vi "MacroGUI_MD.vi"() -> ()   [LabVIEW 2012]
uses:
  Custom Controls and Typedefs/Available Operations Tree.ctl
  Custom Controls and Typedefs/Edit Button.ctl
  Custom Controls and Typedefs/Delete Button.ctl
  Custom Controls and Typedefs/TimeUpdate.ctl
  Custom Controls and Typedefs/Macro_MD_UI Control Refnums.ctl
  Custom Controls and Typedefs/MacroExecutionStates.ctl
  SubVIs/FGV_MacroGen_Commands.ctl
  Custom Controls and Typedefs/Macro_CommandStruct.ctl
  Custom Controls and Typedefs/Macro_Action_List.ctl
  Custom Controls and Typedefs/Macro_ArgumentStruct.ctl
  SubVIs/FormatTree&TableStyle_Commands.ctl
  SubVIs/Timer_MacroGen_Commands.ctl
  <vilib>/Utility/file.llb/Write To Spreadsheet File (string).vi
  GFG/GFG library.lvlib
panel:
  out "Status":string
  out "Index":i32
  out "Timing Data":T1 {"Seconds" scale=0.0..60.0}
  in  "MacroTreeOperation":T4
  in  "File Operation Cluster":cluster{"Load Macro":bool, "SaveAs":bool}
  in  "Table Navigation Cluster":T5
  in  "Parameters":string[][](table)
  in  "Execute Macro":bool
  in  "Add":bool
  in  "Available Actions":T6
  in  "stop":bool
  in  "Macro":string(tree)
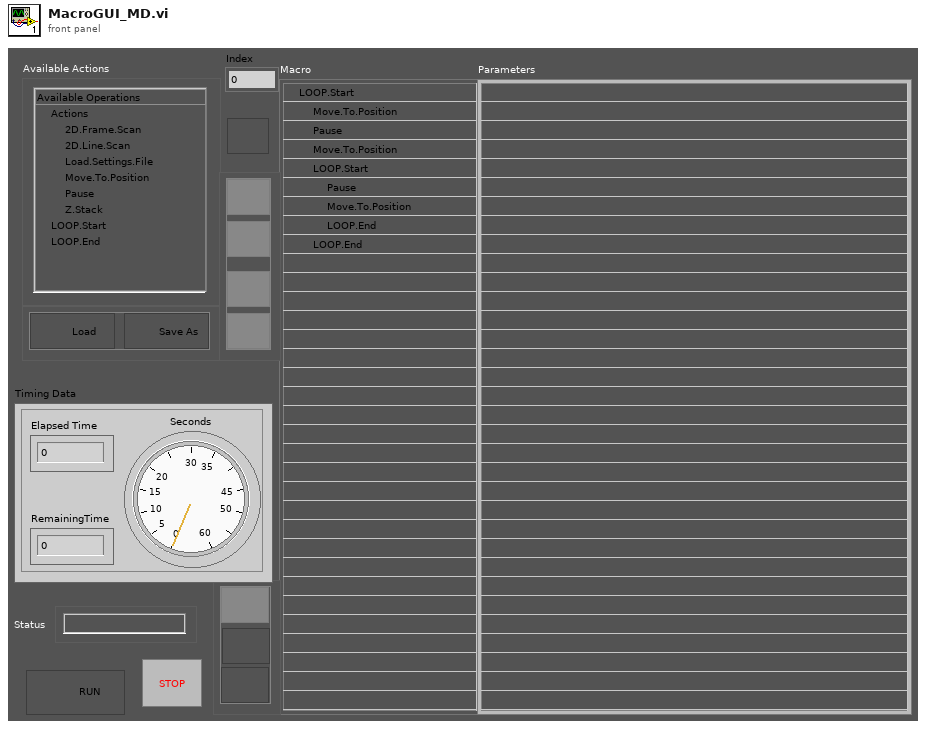
[diagram p1: front panel]
types:
  T1 = typedef "TimeUpdate.ctl" = cluster{"Seconds":dbl, "Elapsed Time":dbl, "RemainingTime":dbl}
  T2 = typedef "Edit Button.ctl" = bool
  T3 = typedef "Delete Button.ctl" = bool
  T4 = cluster{"Save Button":bool, "Edit Button":T2, "Delete Button":T3}
  T5 = cluster{"Table Index Up":bool, "Table Index Up-End":bool, "Table Index Down":bool, "Table Index Down-End":bool}
  T6 = typedef "Available Operations Tree.ctl" = string
  T7 = typedef "MacroExecutionStates.ctl" = enum16{"UI Mode", "Execute Command", "Wait for completion", "Pause"}
  T8 = typedef "Macro_MD_UI Control Refnums.ctl" = cluster{"Available Operations":refnum<vi>, "Created Macro":refnum<vi>, "Indent Item":refnum<vi>, "Add Selected to Macro":refnum<vi>, "Outdent Item":refnum<vi>, "Number of Iterations":refnum<vi>, "Seconds to Wait":refnum<vi>, "Load Macro":refnum<vi>, "Save Macro":refnum<vi>, "Select File to Load":refnum<vi>, "Params Table":refnum<vi>, "Delete":refnum<vi>, "Edit Button":refnum<vi>, "Execute Macro":refnum<vi>}
  T9 = typedef "FGV_MacroGen_Commands.ctl" = enum16{"Initialize", "Get Array", "Load from file", "Insert Item", "Insert at End", "Edit Item", "Delete Item", "Move Items", "Save", "SaveAs"}
  T10 = typedef "FormatTree&TableStyle_Commands.ctl" = enum16{"Colour Row", "Uncolour Row", "Bold Row", "Unbold Row", "Clear", "UpdateVisibleRows"}
  T11 = typedef "Macro_CommandStruct.ctl" = cluster{"Action":T12, "Arguments":T13[]}
  T12 = typedef "Macro_Action_List.ctl" = enum16{"Unknown", "2D.Frame.Scan", "2D.Line.Scan", "Load.Settings.File", "Move.To.Position", "Pause", "Z.Stack", "LOOP.Start", "LOOP.End"}
  T13 = typedef "Macro_ArgumentStruct.ctl" = cluster{"ArgumentName":string, "DataType":enum16{"Numeric", "String"}, "Value":variant}
  T14 = typedef "Timer_MacroGen_Commands.ctl" = enum16{"Start", "Pause", "Run"}
  T15 = cluster{"data name":string, "drag data":variant}[]
  T16 = typedef "LVPoint32TypeDef.ctl" = cluster{"Horizontal":i32, "Vertical":i32}
  T17 = typedef "LVRowAndColumnTypeDef.ctl" = cluster{"Row":i32, "Column":i32}
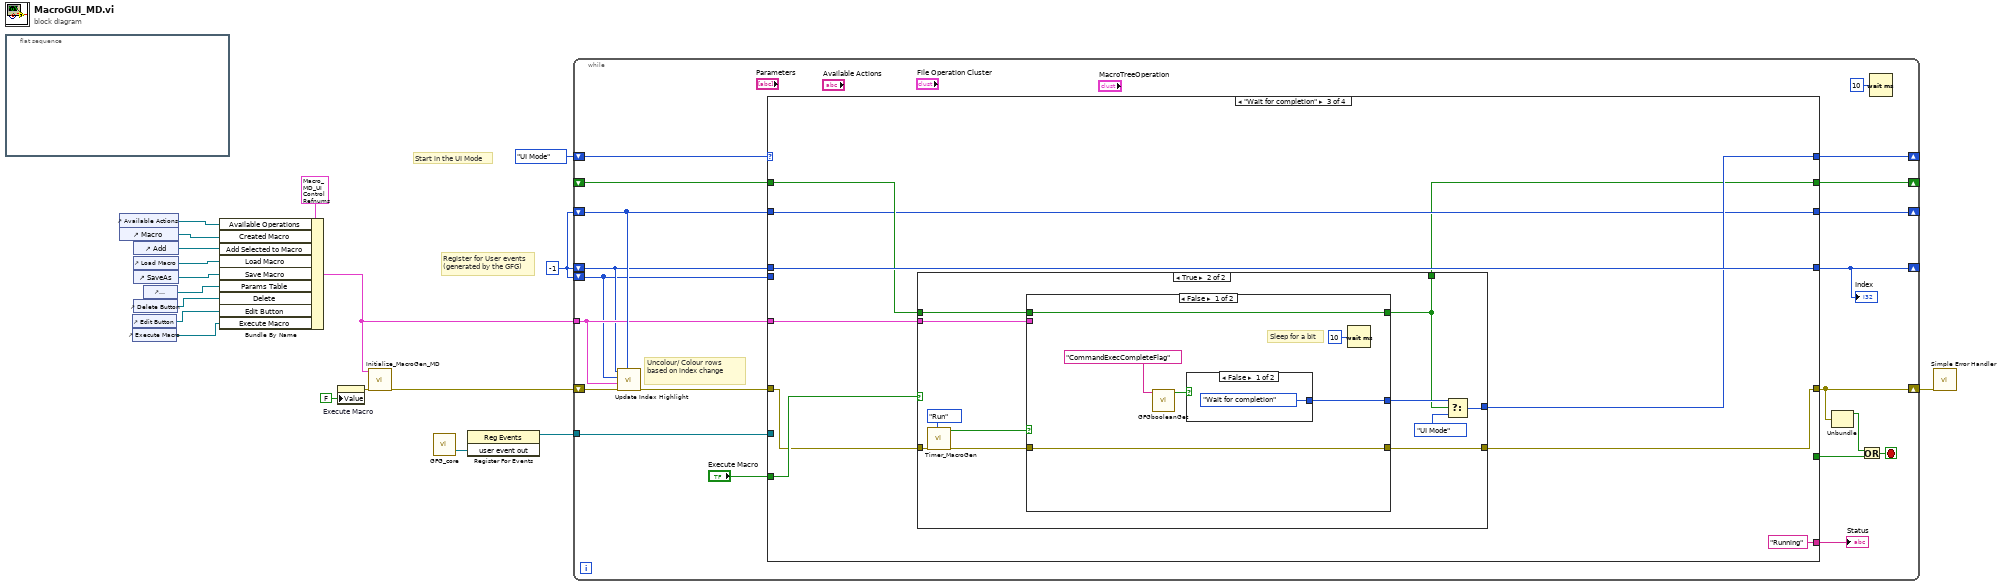
[diagram p0: block diagram]
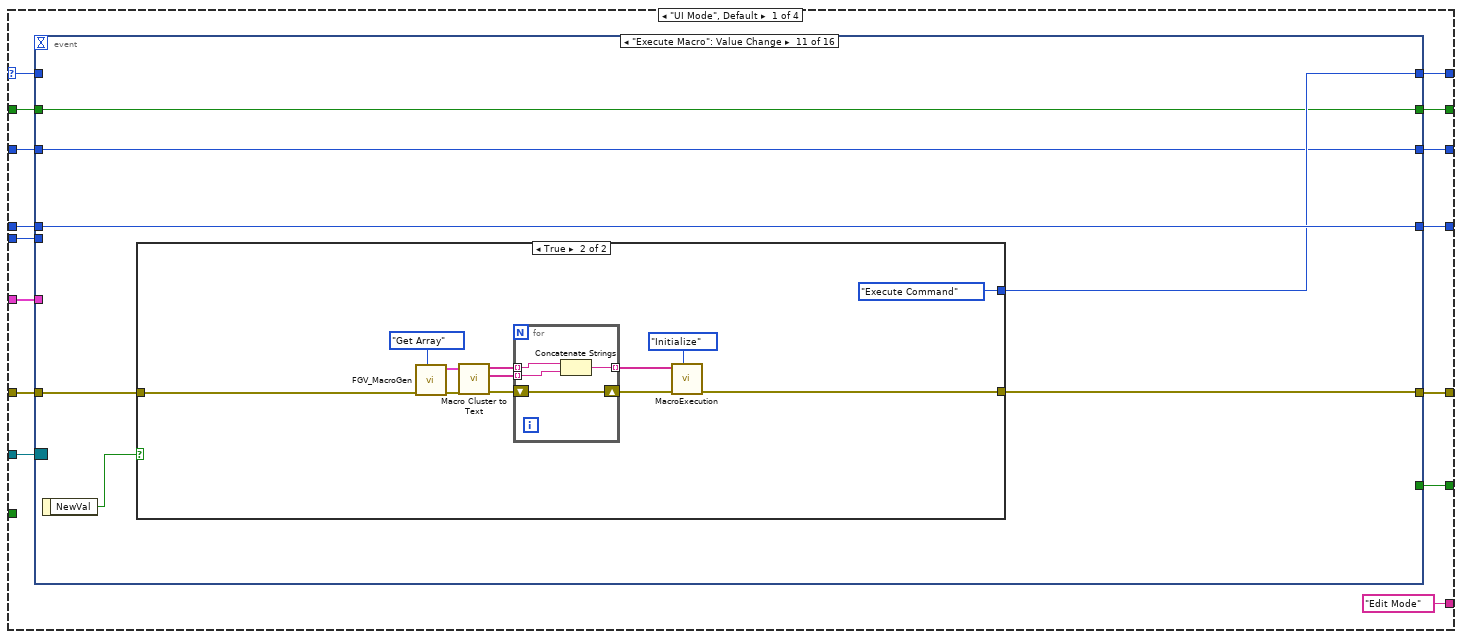
[diagram p2: hidden frame]
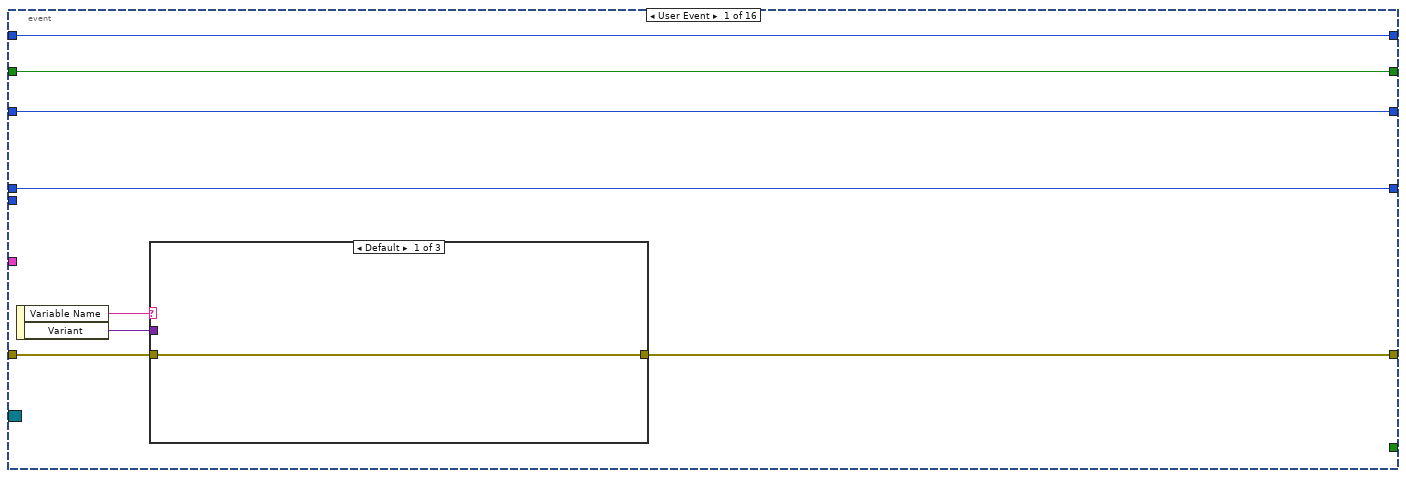
[diagram p3: hidden frame]
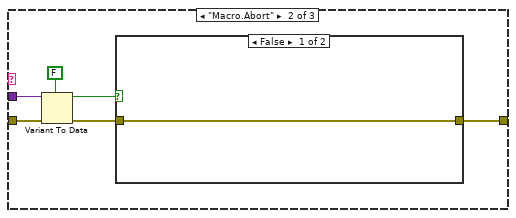
[diagram p4: hidden frame]
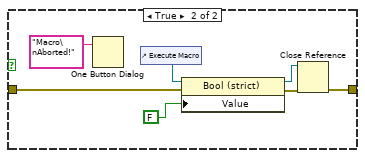
[diagram p5: hidden frame]
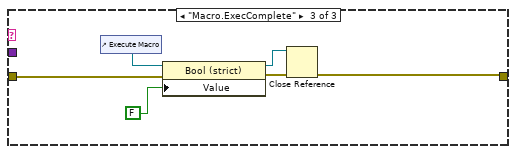
[diagram p6: hidden frame]
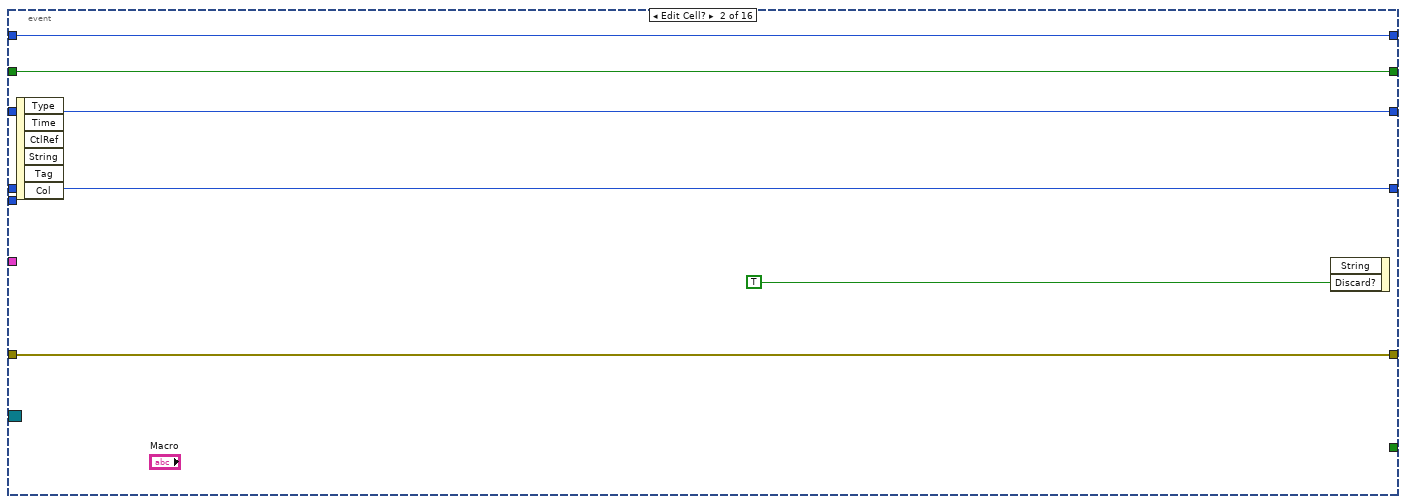
[diagram p7: hidden frame]
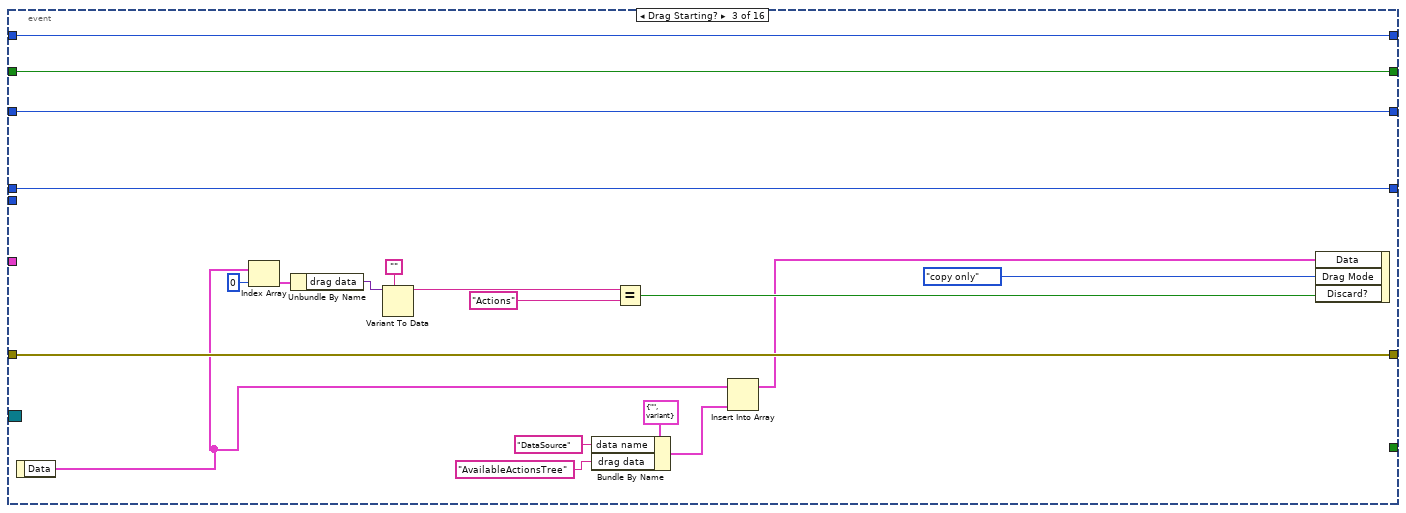
[diagram p8: hidden frame]
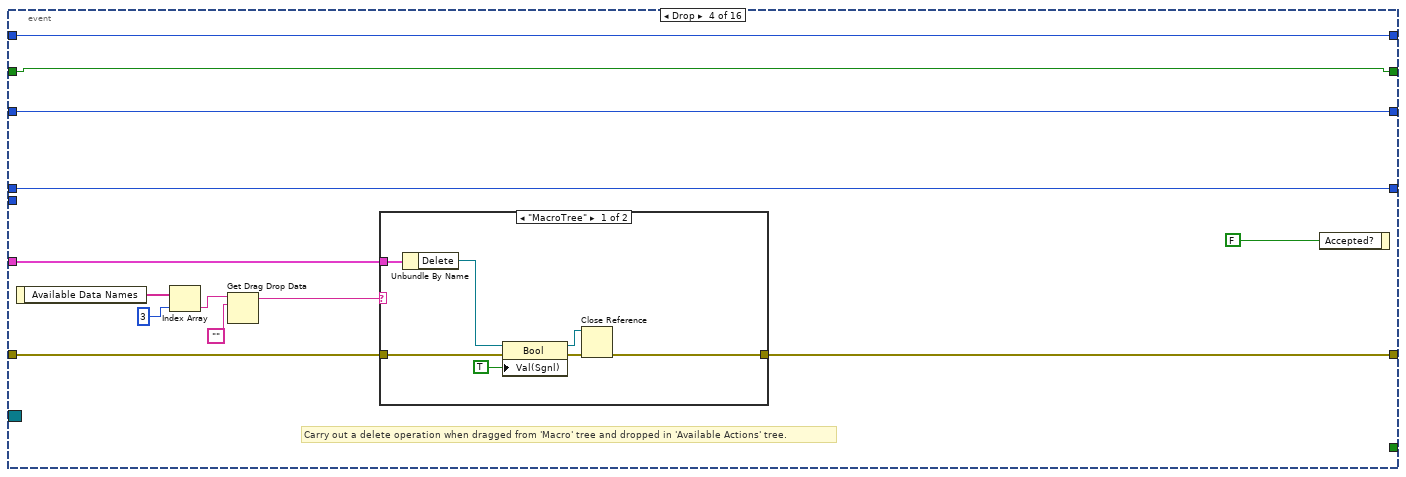
[diagram p9: hidden frame]
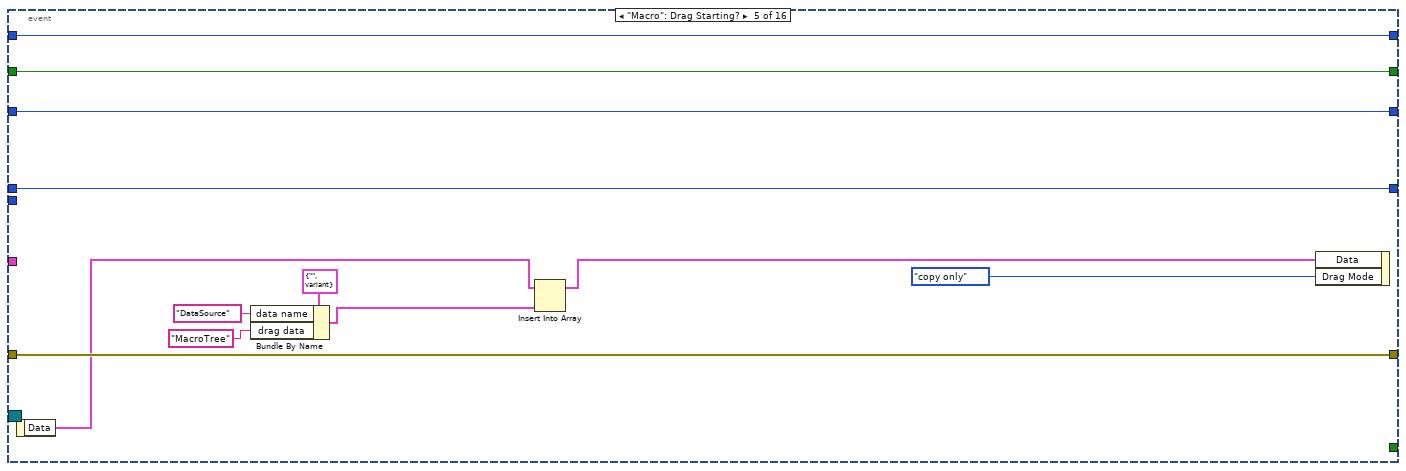
[diagram p11: hidden frame]
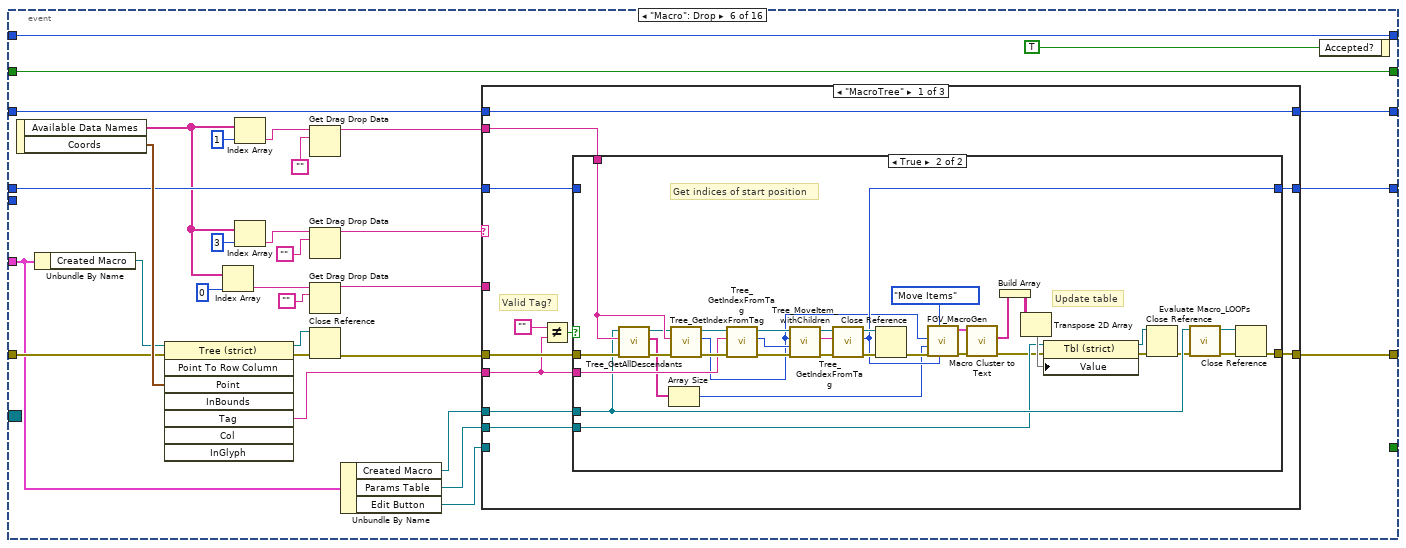
[diagram p12: hidden frame]
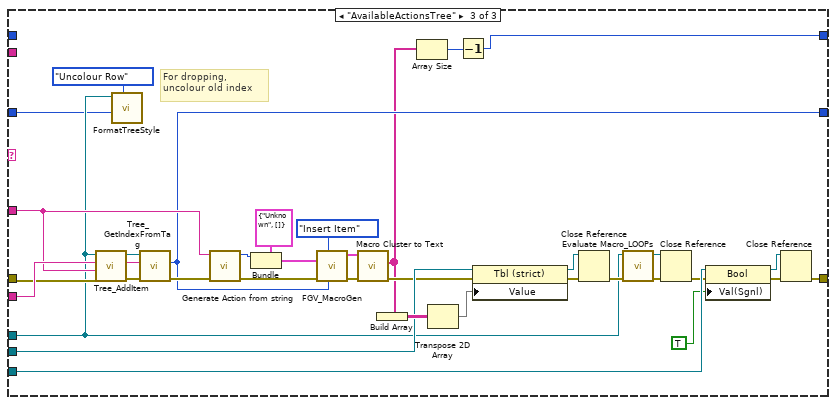
[diagram p15: hidden frame]
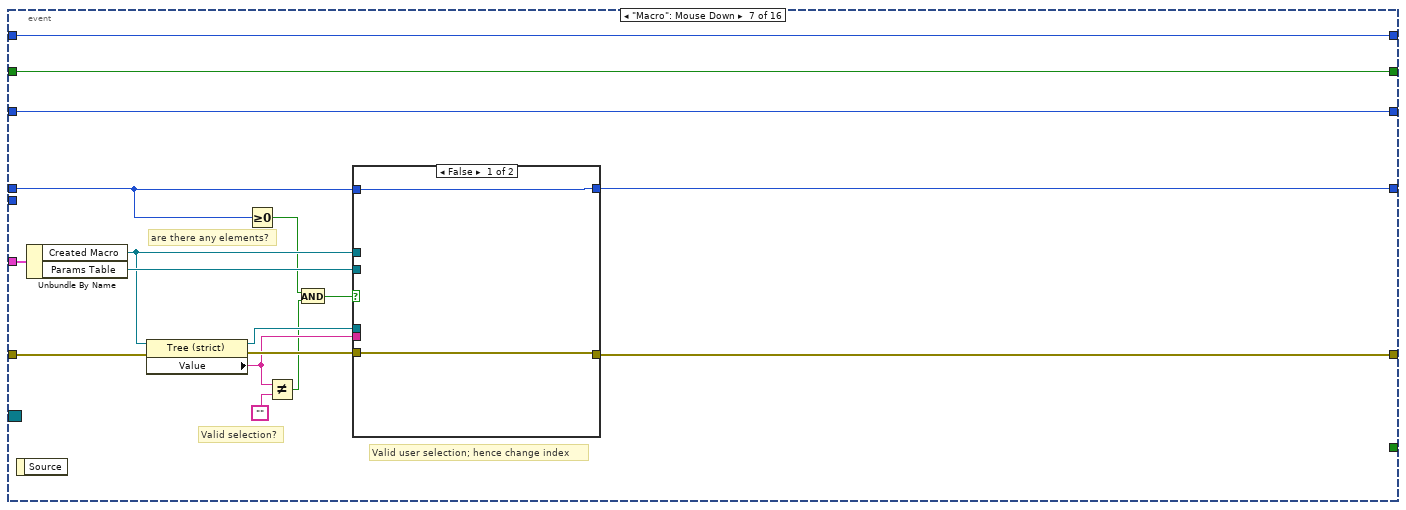
[diagram p16: hidden frame]
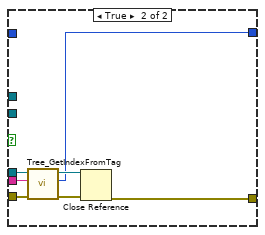
[diagram p17: hidden frame]
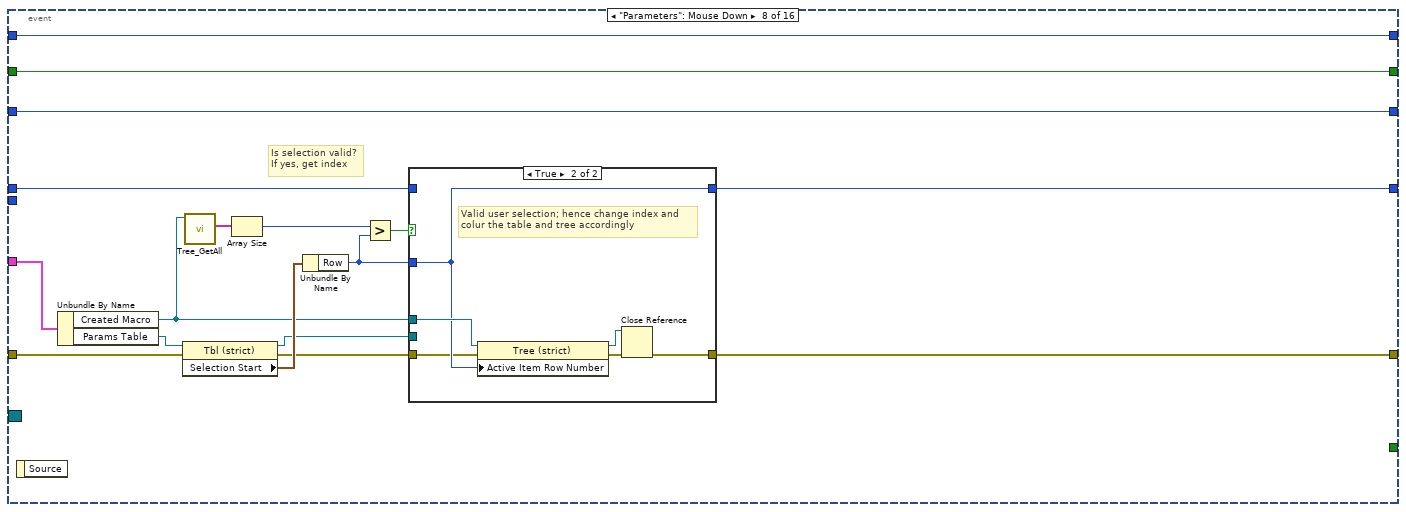
[diagram p18: hidden frame]
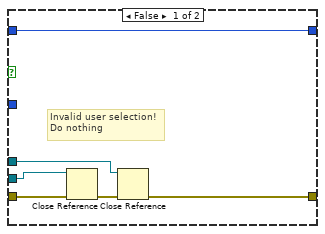
[diagram p19: hidden frame]
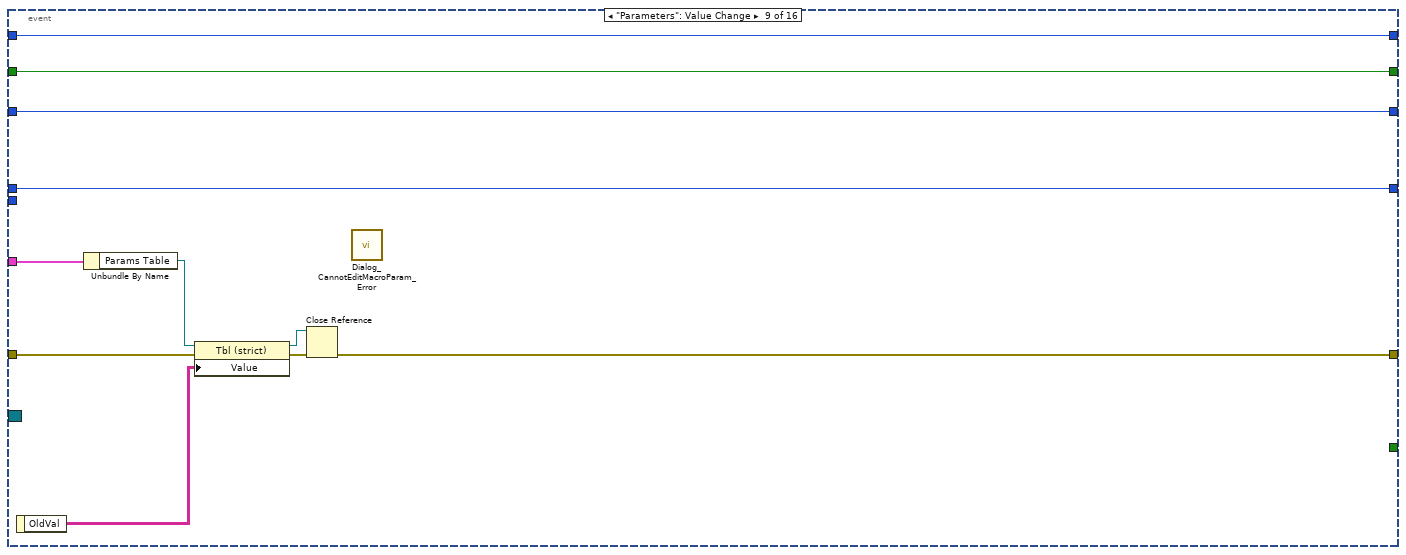
[diagram p20: hidden frame]
diagram:
  w1 = -1 ("Index")
  # "Start in the UI Mode"
  # "Register for User events\n(generated by the GFG)"
  n1 = flat-sequence {
    frame #0 {
    }
  }
  n2 = control-ref of="Available Actions"() -> (w10:refnum<vi>)
  n3 = control-ref of="Macro"() -> (w11:refnum<vi>)
  n4 = control-ref of="Edit Button"() -> (w4:refnum<vi>)
  n5 = control-ref of="Execute Macro"() -> (w2:refnum<vi>)
  n6 = control-ref of="Delete Button"() -> (w5:refnum<vi>)
  n7 = control-ref of="Add"() -> (w17:refnum<vi>)
  n8 = control-ref of="Load Macro"() -> (w16:refnum<vi>)
  n9 = control-ref of="SaveAs"() -> (w15:refnum<vi>)
  n10 = control-ref of="Parameters"() -> (w12:refnum<vi>)
  n11 = Bundle By Name(cluster=T8 {"Available Operations"=refnum, "Created Macro"=refnum, "Indent Item"=refnum, "Add Selected to Macro"=refnum, "Outdent Item"=refnum, "Number of Iterations"=refnum, "Seconds to Wait"=refnum, "Load Macro"=refnum, "Save Macro"=refnum, "Select File to Load"=refnum, "Params Table"=refnum, "Delete"=refnum, "Edit Button"=refnum, "Execute Macro"=refnum} ("UI control refnums"), "Available Operations"=w10, "Created Macro"=w11, "Add Selected to Macro"=w17, "Load Macro"=w16, "Save Macro"=w15, "Params Table"=w12, "Delete"=w5, "Edit Button"=w4, "Execute Macro"=w2) -> (w14:T8)
  n12 = property on="Execute Macro" class="Bool (strict)"("Value"=FALSE ("Execute Macro")) -> (error out=w6:errorcluster)  [unwired: 2 in, 1 out]
  n13 = call "Initialize_MacroGen_MD.vi"("Error In"=w6, "UI control refnums"=w14) -> ("Error Out"=w13:errorcluster)  [unwired: 9 in]
  n14 = call "GFG_core.vi"() -> ("user event out"=w9:refnum<user-event>)  [unwired: 13 in, 6 out]
  n15 = register-events(w9) -> (reference out=w8:refnum<event-registration>)  [unwired: 2 in, 1 out]
  n16 = while {
    tunnel: w14 -> [w22]
    shift-right: [w39] -> w18
    shift-left: w13 -> [w25]
    shift-right: [w27] -> _
    shift-left: w1 -> [w21]
    tunnel: w8 -> [w35]
    shift-right: [w34] -> _
    shift-left: MacroExecutionStates."UI Mode" ("f") -> [w33]
    shift-right: [w30] -> _
    shift-left: _ -> [w29]
    shift-left: w1 -> [w20]
    shift-right: [w28] -> _
    shift-left: w1 -> [w23]
    stop <- w36 stop-if-true
    # "Uncolour/ Colour rows based on index change"
    n17 = call "Update Index Highlight.vi"("Max Index"=w23, "Error In"=w25, "UI control refnums"=w22, "Old Index"=w20, "New Index"=w21) -> ("Error Out"=w24:errorcluster)  [unwired: 6 in]
    n18 = case shown="\"Wait for completion\"" w33 {
      selector: w33 -> [w46 _ _ _]
      tunnel: w22 -> [w54 w586 w651 _]
      tunnel: w24 -> [w53 w593 w649 w707]
      tunnel: [w52 w589 w658 w709] -> w27
      tunnel: w21 -> [w51 w588 w658 w709]
      tunnel: [w50 w592 w655 w704] -> w39
      tunnel: [w49 _ _ _] -> w38
      tunnel: w35 -> [w48 _ _ _]
      tunnel: [w47 w594 w657 w693] -> w34
      tunnel: "Execute Macro" -> [_ w595 w650 w695]
      tunnel: [w44 w590 w652 w708] -> w30
      tunnel: w29 -> [w45 _ w656 w708]
      tunnel: [w43 w587 w654 w696] -> w28
      tunnel: w23 -> [w42 w587 w654 w696]
      tunnel: w20 -> [w41 _ _ _]
      tunnel: ["Edit Mode" w585 "Running" "Running"] -> w26
      frame "UI Mode", Default {
        n19 = event shown="[10] \"Execute Macro\": Value Change" {
          selector: w48 -> [_ _ _ _ _ _ _ _ _ _ _ _ _ _ _ _]
          dyn-events: _ -> [_ _ _ _ _ _ _ _ _ _ _ _ _ _ _ _]
          timeout: _ -> [_ _ _ _ _ _ _ _ _ _ _ _ _ _ _ _]
          tunnel: [_ _ _ _ _ _ _ _ _ _ _ _ _ _ _ "stop"] -> w49
          tunnel: w54 -> [_ _ _ w114 _ w153 w277 w303 w324 w345 _ w424 _ w472 w542 _]
          tunnel: w53 -> [w58 w88 w108 w113 w141 w166 w272 w296 w325 w340 w384 w411 w453 w467 w532 w583]
          tunnel: [w57 w88 w108 w120 w141 w163 w275 w292 w319 w344 w385 w422 w452 w473 w541 w583] -> w50
          tunnel: [w62 w87 w107 w110 w140 w165 w270 w298 w326 w329 w386 w425 w457 w468 w533 w582] -> w52
          tunnel: w51 -> [w62 w87 w107 w110 w140 w154 w267 w299 w326 w343 w386 _ w457 w469 w533 w582]
          tunnel: [w59 w86 w92 w112 w132 w145 w263 w289 w318 w331 w382 w410 w445 w463 w528 w581] -> w47
          tunnel: w46 -> [w59 w86 w92 w112 w132 w145 w263 w289 w318 w331 _ w410 w445 w463 w528 w581]
          tunnel: [w56 w85 w91 w111 w131 w144 w262 w288 w317 w330 w381 w409 w444 w462 w527 w580] -> w44
          tunnel: w45 -> [w56 w85 w91 w111 w131 w144 w262 w288 w317 w330 w381 w409 w444 w462 w527 w580]
          tunnel: [w55 w84 w90 w109 w130 w143 w261 w287 w316 w327 w380 w405 w443 w461 w526 w579] -> w43
          tunnel: w42 -> [w55 w84 w90 w109 w130 w142 w261 w287 w316 w328 w380 _ w443 w460 w526 w579]
          tunnel: w41 -> [_ _ _ _ _ _ _ _ _ _ _ _ _ _ _ _]
          event User Event {
            n20 = event-data() -> ("Variable Name"=w61:string, "Variant"=w60:variant)  [unwired: 1 in]
            n21 = case shown="Default" w61 {
              tunnel: w60 -> [_ w69 _]
              tunnel: w58 -> [w63 w66 w81]
              tunnel: [w63 w64 w78] -> w57
              frame Default {
              }
              frame "Macro.Abort" {
                n22 = Variant To Data(error in=w66, type=FALSE ("Value"), Variant=w69) -> (data=w67:bool, error out=w65:errorcluster)
                n23 = case shown="False" w67 {
                  tunnel: w65 -> [w70 w74]
                  tunnel: [w70 w71] -> w64
                  frame False {
                  }
                  frame True {
                    n24 = One Button Dialog(message="Macro\nAborted!") -> ()  [unwired: 1 in, 1 out]
                    n25 = control-ref of="Execute Macro"() -> (w77:refnum<vi>)
                    n26 = property class="Bool (strict)"(reference=w77, error in=w74, "Value"=FALSE) -> (reference out=w72:refnum<vi>, error out=w73:errorcluster)
                    n27 = Close Reference(reference=w72, error in (no error)=w73) -> (error out=w71:errorcluster)
                  }
                }
              }
              frame "Macro.ExecComplete" {
                n28 = control-ref of="Execute Macro"() -> (w83:refnum<vi>)
                n29 = property class="Bool (strict)"(reference=w83, error in=w81, "Value"=FALSE) -> (reference out=w79:refnum<vi>, error out=w80:errorcluster)
                n30 = Close Reference(reference=w79, error in (no error)=w80) -> (error out=w78:errorcluster)
              }
            }
          }
          event Edit Cell? {
            n31 = event-data() -> ()  [unwired: 1 in, 6 out]
            n32 = event-data("Discard?"=TRUE) -> ()  [unwired: 2 in, 1 out]
          }
          event Drag Starting? {
            n33 = event-data() -> ("Data"=w94:T15)  [unwired: 1 in]
            n34 = Index Array(array=w94, index=0) -> (element=w105:cluster{"data name":string, "drag data":variant})
            n35 = Unbundle By Name(w105) -> ("drag data"=w104:variant)
            n36 = Variant To Data(type="", Variant=w104) -> (data=w102:string)  [unwired: 1 in, 1 out]
            n37 = Bundle By Name(cluster=cluster{"data name":string, "drag data":variant} {"data name"="", "drag data"=variant} ("element"), "data name"="DataSource", "drag data"="AvailableActionsTree" ("data name")) -> (w95:cluster{"data name":string, "drag data":variant})
            n38 = Equal?(x=w102, y="Actions") -> (x = y?=w100:bool)
            n39 = Insert Into Array(array=w94, new element=w95) -> (w93:T15)  [unwired: 1 in]
            n40 = event-data("Data"=w93, "Drag Mode"=enum32{"copy or move", "copy only", "move only"}."copy only", "Discard?"=w100) -> ()  [unwired: 1 in, 1 out]
          }
          event Drop {
            # "Carry out a delete operation when dragged from 'Macro' tree and dropped in 'Available Actions' tree."
            n41 = event-data() -> ("Available Data Names"=w115:string[])  [unwired: 1 in]
            n42 = Index Array(array=w115, index=3) -> (element=w117:string)
            n43 = Get Drag Drop Data(8:"", 9:w117) -> (3:w116:string)  [unwired: 1 in, 1 out]
            n44 = case shown="\"MacroTree\"" w116 {
              tunnel: w113 -> [w126 w129]
              tunnel: [w122 w129] -> w120
              tunnel: w114 -> [w128 _]
              frame "MacroTree" {
                n45 = Unbundle By Name(w128) -> ("Delete"=w127:refnum<vi>)
                n46 = property class="Bool"(reference=w127, error in=w126, "Val(Sgnl)"=TRUE) -> (reference out=w123:refnum<vi>, error out=w124:errorcluster)
                n47 = Close Reference(reference=w123, error in (no error)=w124) -> (error out=w122:errorcluster)
              }
              frame Default {
              }
            }
            n48 = event-data("Accepted?"=FALSE) -> ()  [unwired: 1 in, 1 out]
          }
          event "Macro": Drag Starting? {
            n49 = event-data() -> ("Data"=w138:T15)  [unwired: 1 in]
            n50 = Bundle By Name(cluster=cluster{"data name":string, "drag data":variant} {"data name"="", "drag data"=variant} ("element"), "data name"="DataSource", "drag data"="MacroTree" ("data name")) -> (w133:cluster{"data name":string, "drag data":variant})
            n51 = Insert Into Array(array=w138, new element=w133) -> (w137:T15)  [unwired: 1 in]
            n52 = event-data("Data"=w137, "Drag Mode"=enum32{"copy or move", "copy only", "move only"}."copy only") -> ()  [unwired: 1 in, 1 out]
          }
          event "Macro": Drop {
            n53 = event-data() -> ("Available Data Names"=w147:string[], "Coords"=w169:T16)  [unwired: 1 in]
            n54 = Unbundle By Name(w153) -> ("Created Macro"=w168:refnum<vi>)
            n55 = invoke class="Tree (strict)" method="Point To Row Column"(reference=w168, error in=w166, "Point"=w169) -> (reference out=w149:refnum<vi>, error out=w150:errorcluster, "Tag"=w167:string)  [unwired: 5 in, 5 out]
            n56 = Index Array(array=w147, index=0) -> (element=w171:string)
            n57 = Index Array(array=w147, index=1) -> (element=w158:string)
            n58 = Index Array(array=w147, index=3) -> (element=w160:string)
            n59 = Get Drag Drop Data(8:"", 9:w158) -> (3:w155:string)  [unwired: 1 in, 1 out]
            n60 = Get Drag Drop Data(8:"", 9:w160) -> (3:w159:string)  [unwired: 1 in, 1 out]
            n61 = Get Drag Drop Data(8:"", 9:w171) -> (3:w164:string)  [unwired: 1 in, 1 out]
            n62 = Close Reference(reference=w149, error in (no error)=w150) -> (error out=w148:errorcluster)
            n63 = Unbundle By Name(w153) -> ("Created Macro"=w152:refnum<vi>, "Params Table"=w151:refnum<vi>, "Edit Button"=w146:refnum<vi>)
            n64 = case shown="\"MacroTree\"" w159 {
              tunnel: w167 -> [w176 _ w260]
              tunnel: [w181 w224 w255] -> w165
              tunnel: w148 -> [w184 w223 w233]
              tunnel: w164 -> [_ _ w258]
              tunnel: [w179 w223 w234] -> w163
              tunnel: w155 -> [w183 _ _]
              tunnel: w154 -> [w182 w224 w228]
              tunnel: w152 -> [w178 _ w229]
              tunnel: w151 -> [w180 _ w248]
              tunnel: w146 -> [_ _ w239]
              tunnel: [w174 w222 w225] -> w143
              tunnel: w142 -> [w174 w222 _]
              frame "MacroTree" {
                # "Valid Tag?"
                n65 = Not Equal?(x="", y=w176) -> (x != y?=w177:bool)
                n66 = case shown="True" w177 {
                  tunnel: w184 -> [w185 w206]
                  tunnel: w176 -> [_ w217]
                  tunnel: w183 -> [_ w207]
                  tunnel: w182 -> [w186 _]
                  tunnel: [w186 w199] -> w181
                  tunnel: w180 -> [_ w193]
                  tunnel: [w185 w214] -> w179
                  tunnel: w178 -> [_ w204]
                  frame False {
                  }
                  frame True {
                    # "Update table"
                    # "Get indices of start position"
                    n67 = call "Tree_GetAllDescendants.vi"("Error In"=w206, "Tag"=w207, "Tree Refnum IN"=w204) -> ("Error Out"=w205:errorcluster, "All Descendants"=w202:string[], "Tree Refnum OUT"=w203:refnum<vi>)  [unwired: 6 in]
                    n68 = Array Size(array=w202) -> (size(s)=w197:i32)
                    n69 = call "Tree_GetIndexFromTag.vi"("Error In"=w205, "Tag IN"=w207, "Tree Refnum IN"=w203) -> ("Error Out"=w220:errorcluster, "Index OUT"=w198:i32, "Tree Refnum OUT"=w221:refnum<vi>)  [unwired: 6 in]
                    n70 = call "Tree_GetIndexFromTag.vi"("Error In"=w220, "Tag IN"=w217, "Tree Refnum IN"=w221) -> ("Error Out"=w219:errorcluster, "Index OUT"=w216:i32, "Tree Refnum OUT"=w218:refnum<vi>)  [unwired: 6 in]
                    n71 = call "Tree_MoveItem_withChildren.vi"("Error In"=w219, "End Index"=w216, "Start Index"=w198, "Tree Refnum IN"=w218) -> ("Error Out"=w211:errorcluster, "Moved Tag"=w209:string, "Tree Refnum OUT"=w210:refnum<vi>)  [unwired: 5 in]
                    n72 = call "Tree_GetIndexFromTag.vi"("Error In"=w211, "Tag IN"=w209, "Tree Refnum IN"=w210) -> ("Error Out"=w212:errorcluster, "Index OUT"=w199:i32, "Tree Refnum OUT"=w208:refnum<vi>)  [unwired: 6 in]
                    n73 = Close Reference(reference=w208, error in (no error)=w212) -> (error out=w200:errorcluster)
                    n74 = call "FGV_MacroGen.vi"("Final Index"=w199, "MacroFGV_Commands"=FGV_MacroGen_Commands."Move Items", "Error In"=w200, "Length"=w197, "Start Index"=w198) -> ("Error Out"=w191:errorcluster, "Macro Cluster Array"=w192:T11[])  [unwired: 4 in, 1 out]
                    n75 = call "Macro Cluster to Text.vi"("Error In"=w191, "Macro Cluster Array IN"=w192) -> ("Error Out"=w187:errorcluster, "Argument List (Txt)"=w190:string[])  [unwired: 7 in, 1 out]
                    n76 = Build Array(w190) -> (w195:string[][])
                    n77 = Transpose 2D Array(2D array=w195) -> (transposed array=w194:string[][])
                    n78 = property class="Tbl (strict)"(reference=w193, error in=w187, "Value"=w194) -> (reference out=w189:refnum<vi>, error out=w196:errorcluster)
                    n79 = Close Reference(reference=w189, error in (no error)=w196) -> (error out=w188:errorcluster)
                    n80 = call "Evaluate Macro_LOOPs.vi"("Error In"=w188, "Tree Refnum IN"=w204) -> ("Error Out"=w215:errorcluster, "Tree Refnum OUT"=w213:refnum<vi>)  [unwired: 7 in, 1 out]
                    n81 = Close Reference(reference=w213, error in (no error)=w215) -> (error out=w214:errorcluster)
                  }
                }
              }
              frame Default {
              }
              frame "AvailableActionsTree" {
                # "For dropping, uncolour old index"
                n82 = call "Tree_AddItem.vi"("Error In"=w233, "NEW String"=w258, "Tag at add position"=w260, "Tree Refnum"=w229) -> ("Error Out"=w245:errorcluster, "Added Item Tag"=w243:string, "Tree Refnum OUT"=w244:refnum<vi>)  [unwired: 5 in]
                n83 = call "FormatTreeStyle.vi"("Format Command"=FormatTree&TableStyle_Commands."Uncolour Row", "Row Index"=w228, "Tree Refnum"=w229) -> ()  [unwired: 8 in, 1 out]
                n84 = call "Tree_GetIndexFromTag.vi"("Error In"=w245, "Tag IN"=w243, "Tree Refnum IN"=w244) -> ("Error Out"=w256:errorcluster, "Index OUT"=w255:i32)  [unwired: 6 in, 1 out]
                n85 = call "Generate Action from string.vi"("Error In"=w256, "Command Text"=w258) -> ("Error Out"=w257:errorcluster, "Action"=w241:T12)  [unwired: 8 in]
                n86 = Bundle(cluster=T11 {"Action"=enum."Unknown", "Arguments"=[]} ("Macro Commands"), "Action"=w241) -> (w240:T11)  [unwired: 1 in]
                n87 = call "FGV_MacroGen.vi"("Final Index"=w255, "MacroFGV_Commands"=FGV_MacroGen_Commands."Insert Item", "Error In"=w257, "Macro Command IN"=w240) -> ("Error Out"=w249:errorcluster, "Macro Cluster Array"=w250:T11[])  [unwired: 5 in, 1 out]
                n88 = call "Macro Cluster to Text.vi"("Error In"=w249, "Macro Cluster Array IN"=w250) -> ("Error Out"=w232:errorcluster, "Argument List (Txt)"=w226:string[])  [unwired: 7 in, 1 out]
                n89 = Build Array(w226) -> (w252:string[][])
                n90 = Array Size(array=w226) -> (size(s)=w227:i32)
                n91 = Transpose 2D Array(2D array=w252) -> (transposed array=w251:string[][])
                n92 = Decrement(x=w227) -> (x-1=w225:i32)
                n93 = property class="Tbl (strict)"(reference=w248, error in=w232, "Value"=w251) -> (reference out=w253:refnum<vi>, error out=w254:errorcluster)
                n94 = Close Reference(reference=w253, error in (no error)=w254) -> (error out=w231:errorcluster)
                n95 = call "Evaluate Macro_LOOPs.vi"("Error In"=w231, "Tree Refnum IN"=w229) -> ("Error Out"=w247:errorcluster, "Tree Refnum OUT"=w246:refnum<vi>)  [unwired: 7 in, 1 out]
                n96 = Close Reference(reference=w246, error in (no error)=w247) -> (error out=w238:errorcluster)
                n97 = property class="Bool"(reference=w239, error in=w238, "Val(Sgnl)"=TRUE) -> (reference out=w235:refnum<vi>, error out=w236:errorcluster)
                n98 = Close Reference(reference=w235, error in (no error)=w236) -> (error out=w234:errorcluster)
              }
            }
            n99 = event-data("Accepted?"=TRUE) -> ()  [unwired: 1 in, 1 out]
          }
          event "Macro": Mouse Down {
            # "are there any elements?"
            # "Valid selection?"
            # "Valid user selection; hence change index"
            n100 = event-data() -> ()  [unwired: 1 in, 1 out]
            n101 = Unbundle By Name(w277) -> ("Created Macro"=w273:refnum<vi>, "Params Table"=w276:refnum<vi>)
            n102 = property class="Tree (strict)"(reference=w273, error in=w272) -> (reference out=w271:refnum<vi>, error out=w274:errorcluster, "Value"=w269:string)
            n103 = Greater Or Equal To 0?(x=w267) -> (x >= 0?=w266:bool)
            n104 = Not Equal?(x=w269, y="") -> (x != y?=w265:bool)
            n105 = And(x=w266, y=w265) -> (x .and. y?=w264:bool)
            n106 = case shown="False" w264 {
              tunnel: w267 -> [w279 _]
              tunnel: w276 -> [_ _]
              tunnel: [w278 w280] -> w275
              tunnel: w274 -> [w278 w281]
              tunnel: w273 -> [_ _]
              tunnel: w271 -> [_ w282]
              tunnel: w269 -> [_ w283]
              tunnel: [w279 w284] -> w270
              frame False {
              }
              frame True {
                n107 = call "Tree_GetIndexFromTag.vi"("Error In"=w281, "Tag IN"=w283, "Tree Refnum IN"=w282) -> ("Error Out"=w286:errorcluster, "Index OUT"=w284:i32, "Tree Refnum OUT"=w285:refnum<vi>)  [unwired: 6 in]
                n108 = Close Reference(reference=w285, error in (no error)=w286) -> (error out=w280:errorcluster)
              }
            }
          }
          event "Parameters": Mouse Down {
            # "Is selection valid?\nIf yes, get index"
            n109 = event-data() -> ()  [unwired: 1 in, 1 out]
            n110 = Unbundle By Name(w303) -> ("Created Macro"=w290:refnum<vi>, "Params Table"=w297:refnum<vi>)
            n111 = property class="Tbl (strict)"(reference=w297, error in=w296) -> (reference out=w294:refnum<vi>, error out=w293:errorcluster, "Selection Start"=w302:T17)
            n112 = call "Tree_GetAll.vi"("Tree Refnum IN"=w290) -> ("Tags"=w291:string[])  [unwired: 7 in, 3 out]
            n113 = Array Size(array=w291) -> (size(s)=w301:i32)
            n114 = Unbundle By Name(w302) -> ("Row"=w295:i32)
            n115 = Greater?(x=w301, y=w295) -> (0:w300:bool)
            n116 = case shown="True" w300 {
              tunnel: w299 -> [w309 _]
              tunnel: [w309 w314] -> w298
              tunnel: w294 -> [w305 _]
              tunnel: w290 -> [w304 w315]
              tunnel: w295 -> [_ w314]
              tunnel: w293 -> [w308 w310]
              tunnel: [w306 w311] -> w292
              frame False {
                # "Invalid user selection!\nDo nothing"
                n117 = Close Reference(reference=w305, error in (no error)=w308) -> (error out=w307:errorcluster)
                n118 = Close Reference(reference=w304, error in (no error)=w307) -> (error out=w306:errorcluster)
              }
              frame True {
                # "Valid user selection; hence change index and\ncolur the table and tree accordingly"
                n119 = property class="Tree (strict)"(reference=w315, error in=w310, "Active Item Row Number"=w314) -> (reference out=w312:refnum<vi>, error out=w313:errorcluster)
                n120 = Close Reference(reference=w312, error in (no error)=w313) -> (error out=w311:errorcluster)
              }
            }
          }
          event "Parameters": Value Change {
            n121 = event-data() -> ("OldVal"=w322:string[][])  [unwired: 1 in]
            n122 = Unbundle By Name(w324) -> ("Params Table"=w323:refnum<vi>)
            n123 = property class="Tbl (strict)"(reference=w323, error in=w325, "Value"=w322) -> (reference out=w320:refnum<vi>, error out=w321:errorcluster)
            n124 = Close Reference(reference=w320, error in (no error)=w321) -> (error out=w319:errorcluster)
            n125 = call "Dialog_CannotEditMacroParam_Error.vi"() -> ()  [unwired: 12 in]
          }
          event "Add": Value Change {
            # "Valid Action selected?"
            n126 = event-data() -> ()  [unwired: 1 in, 1 out]
            n127 = Unbundle By Name(w345) -> ("Edit Button"=w332:refnum<vi>, "Created Macro"=w333:refnum<vi>, "Params Table"=w342:refnum<vi>, "Available Operations"=w341:refnum<vi>)
            n128 = property class="Tree (strict)"(reference=w341, error in=w340) -> (reference out=w336:refnum<vi>, error out=w337:errorcluster, "Value"=w334:string)
            n129 = Close Reference(reference=w336, error in (no error)=w337) -> (error out=w335:errorcluster)
            n130 = Not Equal?(x=w334, y="") -> (x != y?=w338:bool)
            n131 = case shown="False" w338 {
              tunnel: [w348 w349] -> w329
              tunnel: [w347 w352] -> w344
              tunnel: w343 -> [w348 _]
              tunnel: w342 -> [_ w373]
              tunnel: w335 -> [w347 w379]
              tunnel: w334 -> [_ w376]
              tunnel: w333 -> [_ w366]
              tunnel: w332 -> [_ w358]
              tunnel: w328 -> [w346 _]
              tunnel: [w346 w349] -> w327
              frame False {
              }
              frame True {
                # "If there is any new data added, increment index"
                n132 = call "Generate Action from string.vi"("Error In"=w379, "Command Text"=w376) -> ("Error Out"=w377:errorcluster, "Action"=w360:T12)  [unwired: 8 in]
                n133 = Bundle By Name(cluster=T11 {"Action"=enum."Unknown", "Arguments"=[]} ("Macro Commands"), "Action"=w360) -> (w359:T11)
                n134 = call "FGV_MacroGen.vi"("MacroFGV_Commands"=FGV_MacroGen_Commands."Insert at End", "Error In"=w377, "Macro Command IN"=w359) -> ("Error Out"=w375:errorcluster, "Macro Cluster Array"=w351:T11[])  [unwired: 6 in, 1 out]
                n135 = Array Size(array=w351) -> (size(s)=w350:i32)
                n136 = call "Tree_AddItem.vi"("Error In"=w375, "NEW String"=w376, "Tree Refnum"=w366) -> ("Error Out"=w374:errorcluster)  [unwired: 6 in, 2 out]
                n137 = Decrement(x=w350) -> (x-1=w349:i32)
                n138 = call "Macro Cluster to Text.vi"("Error In"=w374, "Macro Cluster Array IN"=w351) -> ("Error Out"=w371:errorcluster, "Argument List (Txt)"=w372:string[])  [unwired: 7 in, 1 out]
                n139 = Build Array(w372) -> (w368:string[][])
                n140 = Transpose 2D Array(2D array=w368) -> (transposed array=w367:string[][])
                n141 = property class="Tbl (strict)"(reference=w373, error in=w371, "Value"=w367) -> (reference out=w369:refnum<vi>, error out=w370:errorcluster)
                n142 = Close Reference(reference=w369, error in (no error)=w370) -> (error out=w354:errorcluster)
                n143 = property class="Tree (strict)"(reference=w366, error in=w354, "Active Item Row Number"=w349) -> (reference out=w364:refnum<vi>, error out=w365:errorcluster)
                n144 = call "Evaluate Macro_LOOPs.vi"("Error In"=w365, "Tree Refnum IN"=w364) -> ("Error Out"=w363:errorcluster, "Tree Refnum OUT"=w362:refnum<vi>)  [unwired: 7 in, 1 out]
                n145 = Close Reference(reference=w362, error in (no error)=w363) -> (error out=w353:errorcluster)
                n146 = property class="Bool"(reference=w358, error in=w353, "Val(Sgnl)"=TRUE) -> (reference out=w355:refnum<vi>, error out=w356:errorcluster)
                n147 = Close Reference(reference=w355, error in (no error)=w356) -> (error out=w352:errorcluster)
              }
            }
          }
          event "Execute Macro": Value Change {
            n148 = event-data() -> ("NewVal"=w383:bool)  [unwired: 1 in]
            n149 = case shown="True" w383 {
              tunnel: [w387 w390] -> w385
              tunnel: w384 -> [w387 w389]
              tunnel: [MacroExecutionStates."UI Mode" ("Macro Execution States") MacroExecutionStates."Execute Command" ("Macro Execution States")] -> w382
              frame False {
              }
              frame True {
                n150 = call "FGV_MacroGen.vi"("MacroFGV_Commands"=FGV_MacroGen_Commands."Get Array", "Error In"=w389) -> ("Error Out"=w399:errorcluster, "Macro Cluster Array"=w398:T11[])  [unwired: 7 in, 1 out]
                n151 = call "Macro Cluster to Text.vi"("Error In"=w399, "Macro Cluster Array IN"=w398) -> ("Error Out"=w395:errorcluster, "Argument List (Txt)"=w396:string[], "Action List (Txt)"=w397:string[])  [unwired: 7 in]
                n152 = for {
                  tunnel: w397 -> [w404] mode=indexing
                  tunnel: w396 -> [w403] mode=indexing
                  tunnel: [w402] -> w392 mode=indexing
                  shift-right: [w401] -> w391
                  shift-left: w395 -> [w401]
                  n153 = Concatenate Strings(w404, w403) -> (w402:string)
                }
                n154 = call "MacroExecution.vi"("MacroExecution Command"=enum16{"Initialize", "Run"}."Initialize", "Error In"=w391, "Macro IN"=w392) -> ("Error Out"=w390:errorcluster)  [unwired: 3 in, 5 out]
              }
            }
          }
          event "File Operation Cluster.Load Macro": Value Change {
            w425 = 0 ("Index")
            # "Clear tree first"
            # "Reverse array as items are being added to the top level"
            # "New Index"
            n155 = event-data() -> ()  [unwired: 1 in, 1 out]
            n156 = Unbundle By Name(w424) -> ("Created Macro"=w417:refnum<vi>, "Params Table"=w423:refnum<vi>)
            n157 = call "FGV_MacroGen.vi"("MacroFGV_Commands"=FGV_MacroGen_Commands."Load from file", "Error In"=w411) -> ("Error Out"=w426:errorcluster, "Macro Cluster Array"=w407:T11[])  [unwired: 7 in, 1 out]
            n158 = call "Macro Cluster to Text.vi"("Error In"=w426, "Macro Cluster Array IN"=w407) -> ("Error Out"=w435:errorcluster, "Argument List (Txt)"=w436:string[], "Action List (Txt)"=w419:string[])  [unwired: 7 in]
            n159 = Build Array(w436) -> (w432:string[][])
            n160 = Transpose 2D Array(2D array=w432) -> (transposed array=w431:string[][])
            n161 = Array Size(array=w407) -> (size(s)=w406:i32)
            n162 = property class="Tbl (strict)"(reference=w423, error in=w435, "Value"=w431) -> (reference out=w433:refnum<vi>, error out=w434:errorcluster)
            n163 = Decrement(x=w406) -> (x-1=w405:i32)
            n164 = Close Reference(reference=w433, error in (no error)=w434) -> (error out=w414:errorcluster)
            n165 = invoke class="Tree (strict)" method="Edit Tree Items.Delete"(reference=w417, error in=w414, "tag"="" ("Tag"), "Delete Children"=TRUE ("Delete Children?")) -> (reference out=w412:refnum<vi>, error out=w413:errorcluster)  [unwired: 1 in, 3 out]
            n166 = Reverse 1D Array(array=w419) -> (reversed array=w418:string[])
            n167 = for {
              tunnel: w418 -> [w441] mode=indexing
              shift-right: [w439] -> w421
              shift-left: w413 -> [w440]
              shift-right: [w438] -> w420
              shift-left: w412 -> [w442]
              # "Add items to tree"
              n168 = invoke class="Tree (strict)" method="Edit Tree Items.Add Item"(reference=w442, error in=w440, "Left Cell"=w441) -> (reference out=w438:refnum<vi>, error out=w439:errorcluster)  [unwired: 6 in, 7 out]
            }
            n169 = Close Reference(reference=w420, error in (no error)=w421) -> (error out=w408:errorcluster)
            n170 = property class="Tree (strict)"(reference=w417, error in=w408, "Active Item Row Number"=w425) -> (reference out=w429:refnum<vi>, error out=w430:errorcluster)
            n171 = call "Evaluate Macro_LOOPs.vi"("Error In"=w430, "Tree Refnum IN"=w429) -> ("Error Out"=w428:errorcluster, "Tree Refnum OUT"=w427:refnum<vi>)  [unwired: 7 in, 1 out]
            n172 = Close Reference(reference=w427, error in (no error)=w428) -> (error out=w422:errorcluster)
          }
          event "File Operation Cluster.SaveAs": Value Change {
            n173 = event-data() -> ()  [unwired: 1 in, 1 out]
            n174 = call "FGV_MacroGen.vi"("MacroFGV_Commands"=FGV_MacroGen_Commands."Get Array", "Error In"=w453) -> ("Error Out"=w454:errorcluster, "Macro Cluster Array"=w455:T11[])  [unwired: 7 in, 1 out]
            n175 = call "Macro Cluster to Text.vi"("Error In"=w454, "Macro Cluster Array IN"=w455) -> ("Error Out"=w452:errorcluster, "Argument List (Txt)"=w450:string[], "Action List (Txt)"=w451:string[])  [unwired: 7 in]
            n176 = call "File Dialog"("pattern (all files)"="*.txt") -> ("selected path"=w446:path)  [unwired: 11 in, 3 out]
            n177 = Build Array(w451, w450) -> (w449:string[][])
            n178 = Transpose 2D Array(2D array=w449) -> (transposed array=w448:string[][])
            n179 = call-poly <vilib>:"Write To Spreadsheet File.vi"("2D data"=w448, "file path (dialog if empty)"=w446) -> ()  [unwired: 6 in, 1 out]
          }
          event Value Change {
            n180 = event-data() -> ()  [unwired: 1 in, 4 out]
            n181 = Unbundle By Name(w472) -> ("Created Macro"=w459:refnum<vi>, "Params Table"=w458:refnum<vi>)
            n182 = call "Tree_GetAll.vi"("Error In"=w467, "Tree Refnum IN"=w459) -> ("Error Out"=w466:errorcluster, "Tags"=w465:string[], "Tree Refnum OUT"=w464:refnum<vi>)  [unwired: 6 in, 1 out]
            n183 = Array Size(array=w465) -> (size(s)=w471:i32)
            n184 = Greater Than 0?(x=w471) -> (x > 0?=w470:bool)
            n185 = case shown="True" w470 {
              tunnel: w472 -> [_ _]
              tunnel: w466 -> [w476 w492]
              tunnel: [w476 w485] -> w473
              tunnel: w469 -> [w475 w481]
              tunnel: [w475 w480] -> w468
              tunnel: w464 -> [_ w489]
              tunnel: w458 -> [_ w487]
              tunnel: [w474 w479] -> w461
              tunnel: w460 -> [w474 _]
              frame False {
              }
              frame True {
                # "Get the New Index"
                # "Any more elements?"
                # "Colour row only if there\nare any elements"
                n186 = call "FormatTree&TableStyle.vi"("Format Command"=FormatTree&TableStyle_Commands."Uncolour Row", "Error In"=w492, "Row Index"=w481, "Tbl Refnum"=w487, "Tree Refnum"=w489) -> ("Error Out"=w491:errorcluster)  [unwired: 6 in]
                n187 = call "FGV_MacroGen.vi"("Final Index"=w481, "MacroFGV_Commands"=FGV_MacroGen_Commands."Delete Item", "Error In"=w491) -> ("Error Out"=w497:errorcluster, "Macro Cluster Array"=w495:T11[])  [unwired: 6 in, 1 out]
                n188 = call "Macro Cluster to Text.vi"("Error In"=w497, "Macro Cluster Array IN"=w495) -> ("Error Out"=w504:errorcluster, "Argument List (Txt)"=w505:string[], "Action List (Txt)"=w493:string[])  [unwired: 7 in]
                n189 = Build Array(w505) -> (w503:string[][])
                n190 = Transpose 2D Array(2D array=w503) -> (transposed array=w502:string[][])
                n191 = property class="Tbl (strict)"(reference=w487, error in=w504, "Value"=w502) -> (reference out=w499:refnum<vi>, error out=w500:errorcluster)
                n192 = Array Size(array=w493) -> (size(s)=w496:i32)
                n193 = Decrement(x=w496) -> (x-1=w479:i32)
                n194 = Close Reference(reference=w499, error in (no error)=w500) -> (error out=w498:errorcluster)
                n195 = Greater Or Equal To 0?(x=w479) -> (x >= 0?=w477:bool)
                n196 = property class="Tree"(reference=w489, error in=w498, "Active Item Row Number"=w481) -> (reference out=w509:refnum<vi>, error out=w508:errorcluster)
                n197 = case shown="False" w477 {
                  tunnel: w481 -> [_ w513]
                  tunnel: [-1 ("Index") w512] -> w478
                  frame False {
                  }
                  frame True {
                    n198 = Equal To 0?(x=w513) -> (x = 0?=w514:bool)
                    n199 = case shown="False" w514 {
                      tunnel: w513 -> [w516 _]
                      tunnel: [w515 0 ("Index")] -> w512
                      frame False {
                        n200 = Decrement(x=w516) -> (x-1=w515:i32)
                      }
                      frame True {
                      }
                    }
                  }
                }
                n201 = property class="Tree"(reference=w509, error in=w508) -> (reference out=w490:refnum<vi>, error out=w506:errorcluster, "Active Item Tag"=w507:string)
                n202 = invoke class="Tree" method="Edit Tree Items.Delete"(reference=w490, error in=w506, "tag"=w507, "Delete Children"=FALSE ("Delete Children?")) -> (reference out=w484:refnum<vi>, error out=w488:errorcluster)  [unwired: 1 in, 3 out]
                n203 = case shown="False" w477 {
                  tunnel: w488 -> [w519 w524]
                  tunnel: w478 -> [w518 w520]
                  tunnel: w487 -> [_ w523]
                  tunnel: w484 -> [_ w522]
                  tunnel: [w519 w521] -> w486
                  tunnel: [w518 w520] -> w480
                  frame False {
                    # "Index = 0 if only\n1 element. If no\n elements,\nindex = -1"
                  }
                  frame True {
                    n204 = call "FormatTree&TableStyle.vi"("Format Command"=FormatTree&TableStyle_Commands."Colour Row", "Error In"=w524, "Row Index"=w520, "Tbl Refnum"=w523, "Tree Refnum"=w522) -> ("Error Out"=w521:errorcluster)  [unwired: 6 in]
                  }
                }
                n205 = call "Evaluate Macro_LOOPs.vi"("Error In"=w486, "Tree Refnum IN"=w484) -> ("Error Out"=w483:errorcluster, "Tree Refnum OUT"=w482:refnum<vi>)  [unwired: 7 in, 1 out]
                n206 = Close Reference(reference=w482, error in (no error)=w483) -> (error out=w485:errorcluster)
              }
            }
          }
          event Value Change {
            n207 = event-data() -> ()  [unwired: 1 in, 1 out]
            n208 = Unbundle By Name(w542) -> ("Created Macro"=w534:refnum<vi>)
            n209 = call "Tree_GetTag FromIndex.vi"("Error In"=w532, "Index IN"=w533, "Tree Refnum IN"=w534) -> ("Error Out"=w531:errorcluster, "Tag OUT"=w529:string, "Tree Refnum OUT"=w530:refnum<vi>)  [unwired: 6 in]
            n210 = call "Tree_GetTextFromTag.vi"("Error In"=w531, "Tag IN"=w529, "Tree Refnum IN"=w530) -> ("Error Out"=w537:errorcluster, "String OUT"=w535:string, "Tree Refnum OUT"=w536:refnum<vi>)  [unwired: 6 in]
            n211 = Close Reference(reference=w536, error in (no error)=w537) -> (error out=w538:errorcluster)
            n212 = case shown="\"Pause\"" w535 {
              tunnel: w538 -> [w562 w566 w570 w574 w578]
              tunnel: [w563 w567 w570 w573 w577] -> w543
              tunnel: [w561 w565 T11 {"Action"=enum."Unknown", "Arguments"=[]} ("Macro Commands") w571 w576] -> w540
              tunnel: [w560 w564 TRUE ("Cancelled?") w572 w575] -> w539
              frame "Pause" {
                n213 = call "Dialog_Enter Wait Duration.vi"("Error In"=w562) -> ("Error Out"=w563:errorcluster, "Cancelled?"=w560:bool, "Macro Commands"=w561:T11)  [unwired: 8 in]
              }
              frame "Load.Settings.File" {
                n214 = call "Dialog_Enter Load Setup File Path.vi"("Error In"=w566) -> ("Error Out"=w567:errorcluster, "Cancelled?"=w564:bool, "Macro Commands"=w565:T11)  [unwired: 8 in]
              }
              frame Default {
                # "Do nothing"
              }
              frame "Move.To.Position" {
                n215 = call "Dialog_Enter Stage Position.vi"("Error In"=w574) -> ("Error Out"=w573:errorcluster, "Cancelled?"=w572:bool, "Macro Commands"=w571:T11)  [unwired: 8 in]
              }
              frame "LOOP.Start" {
                n216 = call "Dialog_Enter Loop Iterations.vi"("Error In"=w578) -> ("Error Out"=w577:errorcluster, "Cancelled?"=w575:bool, "Macro Commands"=w576:T11)  [unwired: 8 in]
              }
            }
            n217 = case shown="False" w539 {
              tunnel: w543 -> [w552 w559]
              tunnel: w542 -> [w549 _]
              tunnel: [w547 w559] -> w541
              tunnel: w540 -> [w545 _]
              tunnel: w533 -> [w544 _]
              frame False {
                n218 = call "FGV_MacroGen.vi"("Final Index"=w544, "MacroFGV_Commands"=FGV_MacroGen_Commands."Edit Item", "Error In"=w552, "Macro Command IN"=w545) -> ("Error Out"=w551:errorcluster, "Macro Cluster Array"=w550:T11[])  [unwired: 5 in, 1 out]
                n219 = call "Macro Cluster to Text.vi"("Error In"=w551, "Macro Cluster Array IN"=w550) -> ("Error Out"=w554:errorcluster, "Argument List (Txt)"=w546:string[])  [unwired: 7 in, 1 out]
                n220 = Unbundle By Name(w549) -> ("Params Table"=w548:refnum<vi>)
                n221 = Build Array(w546) -> (w557:string[][])
                n222 = Transpose 2D Array(2D array=w557) -> (transposed array=w558:string[][])
                n223 = property class="Tbl (strict)"(reference=w548, error in=w554, "Value"=w558) -> (reference out=w556:refnum<vi>, error out=w555:errorcluster)
                n224 = Close Reference(reference=w556, error in (no error)=w555) -> (error out=w547:errorcluster)
              }
              frame True {
                # "Cancelled - Do Nothing!"
              }
            }
          }
          event "stop": Value Change {
            n225 = event-data() -> ()  [unwired: 1 in, 1 out]
          }
        }
      }
      frame "Execute Command" {
        n226 = case shown="True" w595 {
          tunnel: [MacroExecutionStates."UI Mode" ("Macro Execution States") w612] -> w594
          tunnel: w593 -> [w598 w611]
          tunnel: [FALSE w605] -> w591
          tunnel: [w598 w607] -> w592
          tunnel: [w597 w606] -> w589
          tunnel: w588 -> [w597 _]
          tunnel: w586 -> [_ w603]
          tunnel: ["Edit Mode" w602] -> w585
          frame False {
            n227 = One Button Dialog(message="Aborted by user!") -> ()  [unwired: 1 in, 1 out]
          }
          frame True {
            n228 = call "MacroExecution.vi"("MacroExecution Command"=enum16{"Initialize", "Run"}."Run", "Error In"=w611) -> ("Error Out"=w610:errorcluster, "Skip?"=w604:bool, "Paused?"=w609:bool, "Execution Complete?"=w605:bool, "Pause Duration"=w608:dbl, "Current Execution Index"=w606:i32)  [unwired: 4 in]
            n229 = case shown="True" w605 {
              tunnel: [w615 MacroExecutionStates."UI Mode" ("Macro Execution States")] -> w612
              tunnel: w610 -> [w620 w643]
              tunnel: w609 -> [w618 _]
              tunnel: w608 -> [w619 _]
              tunnel: [w617 w640] -> w607
              tunnel: w604 -> [w616 _]
              tunnel: w603 -> [_ w646]
              tunnel: ["Running" "Edit Mode"] -> w602
              frame False {
                n230 = case shown="False" w618 {
                  tunnel: [w622 MacroExecutionStates."Pause" ("Macro Execution States")] -> w615
                  tunnel: w619 -> [_ w634]
                  tunnel: w620 -> [w623 w636]
                  tunnel: [w621 w635] -> w617
                  tunnel: w616 -> [w624 _]
                  frame False {
                    n231 = case shown="False" w624 {
                      tunnel: w623 -> [w627 w631]
                      tunnel: [w626 w631] -> w621
                      tunnel: [MacroExecutionStates."Wait for completion" ("Macro Execution States") MacroExecutionStates."Execute Command" ("Macro Execution States")] -> w622
                      frame False {
                        # "Go to 'wait for completion' state"
                        n232 = call "Timer_MacroGen.vi"("Timer Command"=Timer_MacroGen_Commands."Start", "Error In"=w627, "Set Time (ms)"=3000.0) -> ("Error Out"=w626:errorcluster)  [unwired: 5 in, 3 out]
                      }
                      frame True {
                        # "This is a LOOP.Start or LOOP.End, skip to next"
                      }
                    }
                  }
                  frame True {
                    n233 = Multiply(x=1000.0 ("Pause Duration"), y=w634) -> (x*y=w632:dbl)
                    n234 = call "Timer_MacroGen.vi"("Timer Command"=Timer_MacroGen_Commands."Start", "Error In"=w636, "Set Time (ms)"=w632) -> ("Error Out"=w635:errorcluster)  [unwired: 5 in, 3 out]
                  }
                }
              }
              frame True {
                n235 = Unbundle By Name(w646) -> ("Execute Macro"=w645:refnum<vi>)
                n236 = property class="Bool (strict)"(reference=w645, error in=w643, "Value"=FALSE) -> (reference out=w641:refnum<vi>, error out=w642:errorcluster)
                n237 = One Button Dialog(message="Execution Complete!") -> ()  [unwired: 1 in, 1 out]
                n238 = Close Reference(reference=w641, error in (no error)=w642) -> (error out=w640:errorcluster)
              }
            }
          }
        }
        n239 = Not(x=w591) -> (.not. x?=w590:bool)
      }
      frame "Wait for completion" {
        n240 = case shown="True" w650 {
          tunnel: [MacroExecutionStates."UI Mode" ("f") w673] -> w657
          tunnel: w656 -> [_ w664]
          tunnel: [w659 w672] -> w655
          tunnel: w649 -> [w659 w667]
          tunnel: [FALSE w663] -> w652
          tunnel: w651 -> [_ w665]
          frame False {
            # "If timeout, report error and go to UI Mode"
            n241 = One Button Dialog(message="Run aborted by user!") -> ()  [unwired: 1 in, 1 out]
          }
          frame True {
            n242 = call "Timer_MacroGen.vi"("Timer Command"=Timer_MacroGen_Commands."Run", "Error In"=w667) -> ("Error Out"=w666:errorcluster, "Complete?"=w668:bool)  [unwired: 6 in, 2 out]
            n243 = case shown="False" w668 {
              tunnel: [w675 w683] -> w672
              tunnel: w666 -> [w675 w685]
              tunnel: [w676 MacroExecutionStates."UI Mode" ("Macro Execution States")] -> w671
              tunnel: w665 -> [_ w686]
              tunnel: w664 -> [w679 _]
              tunnel: [w679 FALSE] -> w663
              frame False {
                # "Sleep for a bit"
                n244 = call "GFGbooleanGet.vi"("Variable Name in"="CommandExecCompleteFlag") -> ("Boolean"=w677:bool)  [unwired: 10 in]
                n245 = case shown="False" w677 {
                  tunnel: [MacroExecutionStates."Wait for completion" ("Macro Execution States") MacroExecutionStates."Execute Command" ("Macro Execution States")] -> w676
                  frame False {
                  }
                  frame True {
                  }
                }
                n246 = Wait (ms)(milliseconds to wait=u32 10) -> ()  [unwired: 1 out]
              }
              frame True {
                # "If timeout, report error and go to UI Mode"
                n247 = Unbundle By Name(w686) -> ("Execute Macro"=w690:refnum<vi>)
                n248 = property class="Bool (strict)"(reference=w690, error in=w685, "Value"=FALSE) -> (reference out=w687:refnum<vi>, error out=w688:errorcluster)
                n249 = Close Reference(reference=w687, error in (no error)=w688) -> (error out=w683:errorcluster)
                n250 = One Button Dialog(message="Command Timed Out!") -> ()  [unwired: 1 in, 1 out]
              }
            }
            n251 = Select(t=w671, s=w663, f=MacroExecutionStates."UI Mode") -> (s? t:f=w673:T7)
          }
        }
      }
      frame "Pause" {
        w697 = 1000.0 ("Remaining Time (ms)")
        # "Has User aborted the run?"
        # "Next State"
        # "Sleep for a bit to save processor time"
        n252 = event shown="[0] Timeout" {
          selector: _ -> [_]
          dyn-events: _ -> [_]
          timeout: 200 -> [_]
          tunnel: w707 -> [w717]
          tunnel: [w716] -> w705
          tunnel: [w715] -> w704
          tunnel: [w714] -> w701
          tunnel: [w713] -> w700
          event Timeout {
            n253 = event-data() -> ()  [unwired: 1 in, 2 out]
            n254 = call "Timer_MacroGen.vi"("Timer Command"=Timer_MacroGen_Commands."Run", "Error In"=w717) -> ("Error Out"=w715:errorcluster, "Remaining Time (ms)"=w713:dbl, "Elapsed Time (ms)"=w714:dbl, "Complete?"=w716:bool)  [unwired: 6 in]
          }
        }
        n255 = Divide(x=w701, y=w697) -> (x/y=w699:dbl)
        n256 = Divide(x=w700, y=w697) -> (x/y=w698:dbl)
        n257 = Bundle By Name(cluster=T1 {"Seconds"=0.0, "Elapsed Time"=0.0, "RemainingTime"=0.0} ("Timing Data"), "Elapsed Time"=w699, "RemainingTime"=w698) -> (→"Timing Data":T1)
        n258 = case shown="True" w705 {
          tunnel: [MacroExecutionStates."Pause" ("f") MacroExecutionStates."Execute Command" ("f")] -> w694
          frame False {
          }
          frame True {
          }
        }
        n259 = case shown="True" w695 {
          tunnel: w694 -> [_ w712]
          tunnel: [MacroExecutionStates."UI Mode" ("f") w712] -> w693
          frame False {
            n260 = One Button Dialog(message="Aborted!") -> ()  [unwired: 1 in, 1 out]
          }
          frame True {
          }
        }
      }
    }
    "Index" <- w27
    "Status" <- w26
    n261 = Unbundle(w39) -> ("status"=w37:bool)  [unwired: 2 out]
    n262 = Or(x=w37, y=w38) -> (x .or. y?=w36:bool)
    n263 = Wait (ms)(milliseconds to wait=u32 10) -> ()  [unwired: 1 out]
  }
  n264 = call <vilib>:"Simple Error Handler.vi"("error in (no error)"=w18) -> ()  [unwired: 4 in, 5 out]
